vi "STRUCT_3_STAGE_PL.vi"(8 "Dataflow In":errorcluster) -> (0 "Dataflow Out":errorcluster)   [LabVIEW 2019]
panel:
  # "*******************************************************************\nBiogas Plant Control\n\nAuthor: Paul Zügel\nGCSC-Frankfurt am Main 2020\n\n*******************************************************************"
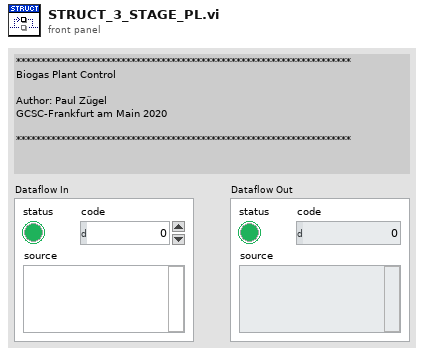
[diagram p1: front panel]
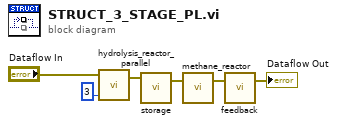
[diagram p0: block diagram]
diagram:
  n1 = call "hydrolysis_reactor_parallel.vi"("Instances"=3, "Dataflow In"="Dataflow In") -> ("Dataflow Out"=w1:errorcluster)  [unwired: 2 in]
  n2 = call "storage.vi"("Dataflow In #1"=w1) -> ("Dataflow Out"=w4:errorcluster)  [unwired: 3 in]
  n3 = call "methane_reactor.vi"("Dataflow In"=w4) -> ("Dataflow Out"=w3:errorcluster)  [unwired: 2 in]
  n4 = call "feedback.vi"("Dataflow In"=w3) -> ("Dataflow Out"=→"Dataflow Out":errorcluster)  [unwired: 2 in]
